vi "Query.vi"(0 "RedPitaya connection in":refnum<k5>, 5 "SCPI Query":string="ACQ:BUF:SIZE?", 9 "timeout ms (2000)":i32=2000, 11 "error in":errorcluster) -> (4 "RedPitaya connection out":refnum<k5>, 6 "data out":string, 15 "error out":errorcluster)   [LabVIEW 2010, in "RedPitaya.lvlib"]
doc: "Sends <b>SCPI Query</b> to pitaya and outputs response on <b>data out</b>."
uses:
  RedPitaya.lvlib
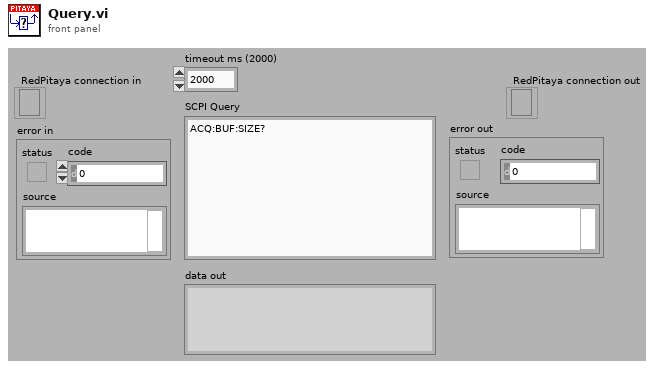
[diagram p1: front panel]
types:
  T1 = enum16{"Standard", "Buffered", "CRLF", "Immediate"}
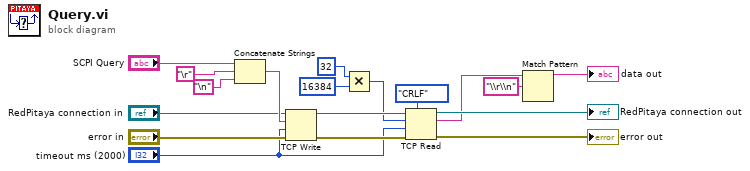
[diagram p0: block diagram]
diagram:
  n1 = Concatenate Strings("SCPI Query", "\r", "\n") -> (w11:string)
  n2 = TCP Write(connection ID="RedPitaya connection in", data in=w11, error in (no error)="error in", 9:"timeout ms (2000)") -> (connection ID out=w18:refnum<k5>, error out=w17:errorcluster)  [unwired: 1 out]
  n3 = Multiply(x=32, y=16384 ("bytes to read")) -> (x*y=w5:i32)
  n4 = TCP Read(connection ID=w18, bytes to read=w5, error in (no error)=w17, 7:T1."CRLF" ("mode (standard)"), 9:"timeout ms (2000)") -> (connection ID out=→"RedPitaya connection out":refnum<k5>, data out=w4:string, error out=→"error out":errorcluster)
  n5 = Match Pattern(string=w4, regular expression="\\r\\n") -> (before substring=→"data out":string)  [unwired: 1 in, 3 out]
